vi "SCT Merge Filter.vi"(9 "Columns to Merge":string[](array[string]), 10 "Attributes":string[](array[string]), 11 "Filter Config":cluster{"Attributes":string, "Display":bool}[](array[cluster])) -> (3 "Merged Filter Config":cluster{"Attributes":string, "Display":bool}[](array[cluster]))   [LabVIEW 2016]
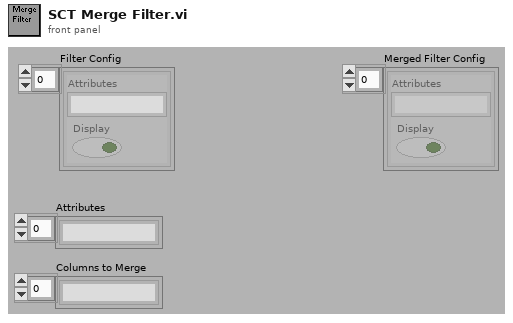
[diagram p1: front panel]
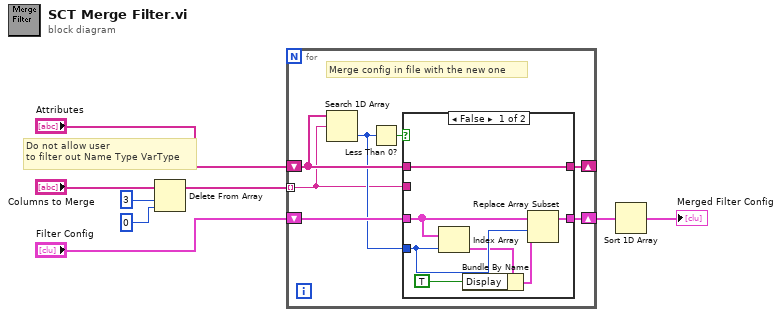
[diagram p0: block diagram]
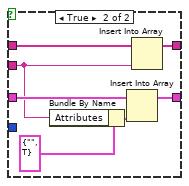
[diagram p2: hidden frame]
diagram:
  # "Do not allow user\nto filter out Name Type VarType"
  n1 = Delete From Array(array="Columns to Merge", length=3, index=0) -> (array with subset deleted=w3:string[])  [unwired: 1 out]
  n2 = for {
    tunnel: w3 -> [w9] mode=indexing
    shift-right: [w13] -> _
    shift-left: "Attributes" -> [w15]
    shift-right: [w10] -> w5
    shift-left: "Filter Config" -> [w12]
    # "Merge config in file with the new one"
    n3 = Search 1D Array(1D array=w15, element=w9) -> (index of element=w11:i32)  [unwired: 1 in]
    n4 = Less Than 0?(x=w11) -> (x < 0?=w14:bool)
    n5 = case shown="False" w14 {
      tunnel: w15 -> [w22 w29]
      tunnel: [w22 w28] -> w13
      tunnel: w12 -> [w21 w27]
      tunnel: w11 -> [w19 _]
      tunnel: [w20 w26] -> w10
      tunnel: w9 -> [_ w23]
      frame False {
        n6 = Index Array(array=w21, index=w19) -> (element=w18:cluster{"Attributes":string, "Display":bool})
        n7 = Bundle By Name(cluster=w18, "Display"=TRUE) -> (w16:cluster{"Attributes":string, "Display":bool})
        n8 = Replace Array Subset(array=w21, new element=w16, index=w19) -> (w20:cluster{"Attributes":string, "Display":bool}[])
      }
      frame True {
        n9 = Bundle By Name(cluster=cluster{"Attributes":string, "Display":bool} {"Attributes"="", "Display"=TRUE} ("new element/subarray"), "Attributes"=w23) -> (w24:cluster{"Attributes":string, "Display":bool})
        n10 = Insert Into Array(array=w27, new element=w24) -> (w26:cluster{"Attributes":string, "Display":bool}[])  [unwired: 1 in]
        n11 = Insert Into Array(array=w29, new element=w23) -> (w28:string[])  [unwired: 1 in]
      }
    }
  }
  n12 = Sort 1D Array(array=w5) -> (sorted array=→"Merged Filter Config":cluster{"Attributes":string, "Display":bool}[])
